vi "Construct_Remaining_Subtrack_101_More_2_Subtrks-1.vi"(0 "[IN] Still connected\ntracks in group":T2, 1 "[IN] Indexes for Jumps":i32[](array[numeric]), 5 "[IN] Clusters for Re\nconstructed Tracks":T1, 7 "[IN] Index of recon\nstructed tracks":i32, 11 "error IN":errorcluster, 12 "[IN] # column of re\nmaining elongation":i32, 13 "[IN] Indicies of Po\nints Inside Trks":i32[](array[numeric]), 14 "[IN] Indicies of all \nAffected Tracks \n(initial point = 0)":i32[](array[numeric])) -> (6 "[OUT] Clusters for Re\nconstructed Tracks":T1, 15 "error OUT":errorcluster)   [LabVIEW 2017]
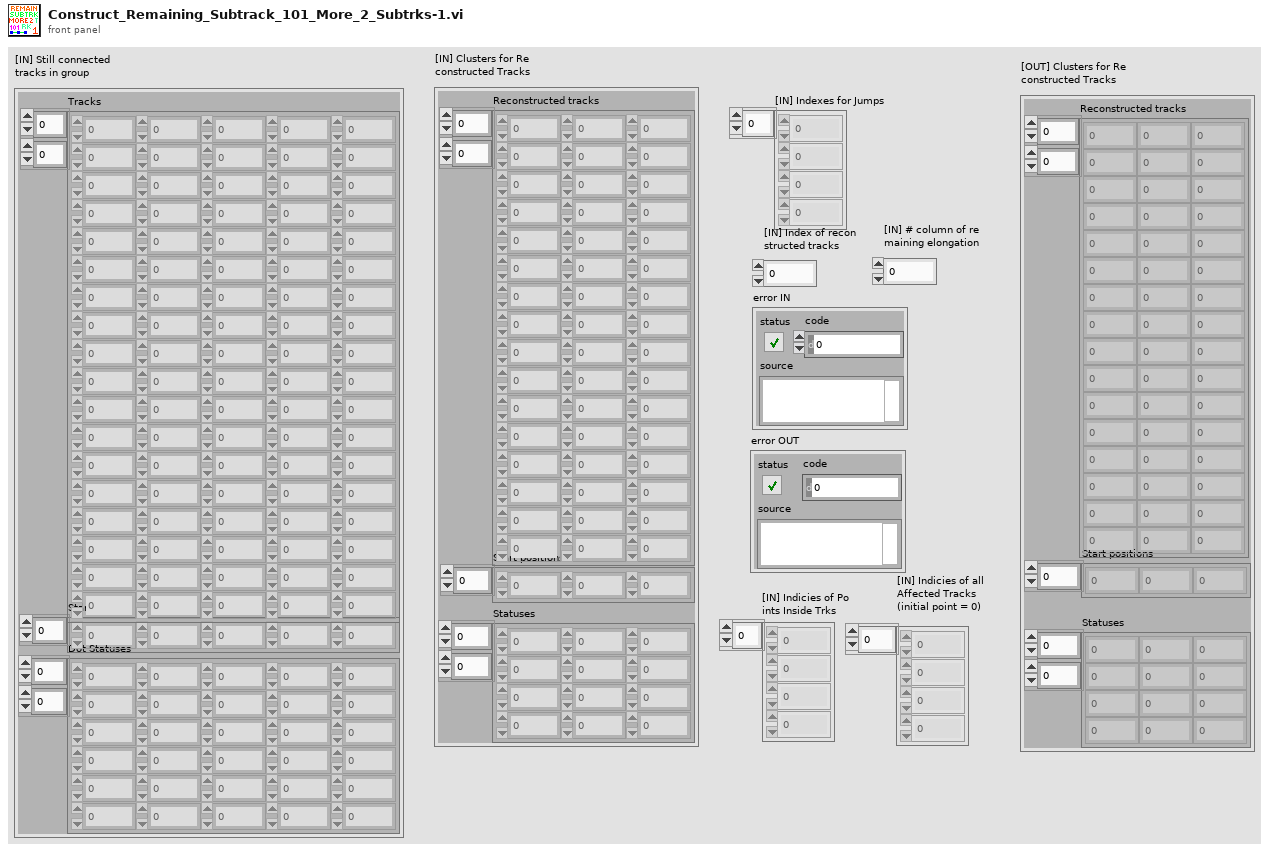
[diagram p1: front panel]
types:
  T1 = cluster{"Reconstructed tracks":dbl[][], "Start positions":i32[], "Statuses":i16[][]}
  T2 = cluster{"Tracks":dbl[][], "Start Pos":i32[], "Dot Statuses":i16[][]}
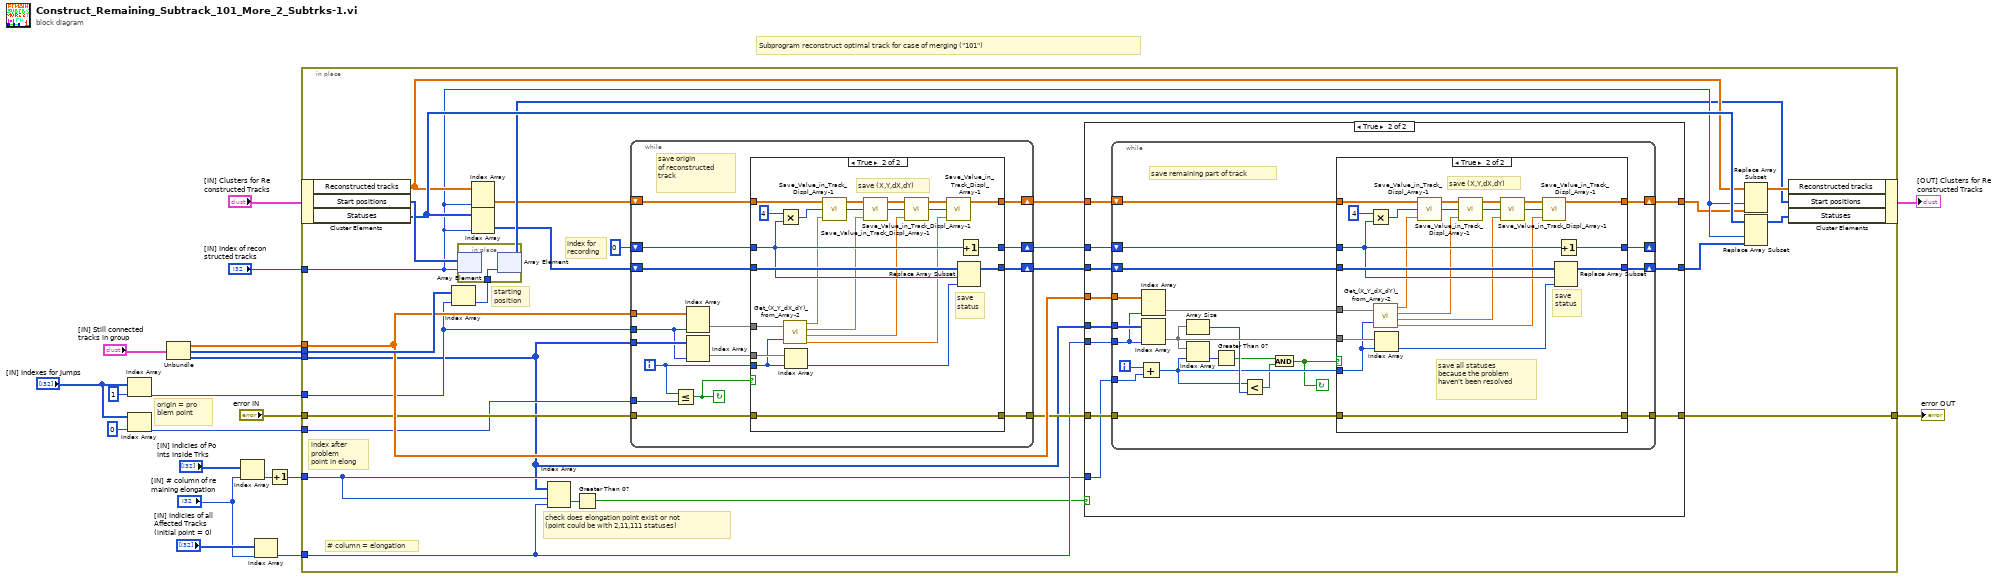
[diagram p0: block diagram]
diagram:
  # "origin = pro\nblem point"
  # "Subprogram reconstruct optimal track for case of merging (\"101\")"
  n1 = Index Array(array="[IN] Indexes for Jumps", index=1) -> (element=w14:i32)
  n2 = Index Array(array="[IN] Indexes for Jumps", index=0) -> (element=w10:i32)
  n3 = Unbundle("[IN] Still connected\ntracks in group") -> ("Tracks"=w11:dbl[][], "Start Pos"=w12:i32[], "Dot Statuses"=w13:i16[][])
  n4 = Index Array(array="[IN] Indicies of Po\nints Inside Trks", index="[IN] # column of re\nmaining elongation") -> (element=w3:i32)
  n5 = Index Array(array="[IN] Indicies of all \nAffected Tracks \n(initial point = 0)", index="[IN] # column of re\nmaining elongation") -> (element=w5:i32)
  n6 = Increment(x=w3) -> (x+1=w2:i32)
  n7 = in-place {
    in-place-border: "[IN] Index of recon\nstructed tracks" -> [w43]
    in-place-border: w14 -> [w25]
    in-place-border: w13 -> [w21]
    in-place-border: w12 -> [w48]
    in-place-border: w11 -> [w47]
    in-place-border: w10 -> [w24]
    in-place-border: "error IN" -> [w42]
    in-place-border: w5 -> [w27]
    in-place-border: [w38] -> w7
    in-place-border: w2 -> [w26]
    # "check does elongation point exist or not  \n(point could be with 2,11,111 statuses)"
    # "# column = elongation"
    # "index after\nproblem \npoint in elong"
    # "index for\nrecording"
    # "starting\nposition"
    n8 = in-place-cluster #1("[IN] Clusters for Re\nconstructed Tracks") -> ("Reconstructed tracks"=w44:dbl[][], "Start positions"=w46:i32[], "Statuses"=w45:i16[][])
    n9 = Index Array(array=w48, index=w25) -> (element=w37:i32)
    n10 = in-place {
      in-place-border: w37 -> [w154]
      n11 = in-place-array #2(w46, w43) -> ()  [unwired: 1 out]
      n12 = in-place-array #2(w154) -> (w40:i32[])  [unwired: 1 out]
    }
    n13 = Index Array(array=w44, index (col)=w43) -> (element=w35:dbl[])  [unwired: 1 in]
    n14 = Index Array(array=w45, index (col)=w43) -> (element=w34:i16[])  [unwired: 1 in]
    n15 = Index Array(array=w21, index (row)=w26, index (col)=w27) -> (element=w23:i16)
    n16 = Greater Than 0?(x=w23) -> (x > 0?=w22:bool)
    n17 = while {
      tunnel: w24 -> [w113]
      tunnel: w47 -> [w126]
      tunnel: w21 -> [w125]
      tunnel: w25 -> [w124]
      shift-right: [w118] -> w33
      shift-left: w35 -> [w123]
      shift-right: [w116] -> w31
      shift-left: w34 -> [w120]
      shift-right: [w117] -> w32
      shift-left: 0 -> [w119]
      tunnel: w42 -> [w111]
      tunnel: [w115] -> w30
      i -> [w114]
      stop <- w112 continue-if-true
      # "save origin \nof reconstructed \ntrack"
      n18 = Less Or Equal?(x=w114, y=w113) -> (x <= y?=w112:bool)
      n19 = Index Array(array=w126, index (col)=w124) -> (element=w122:dbl[])  [unwired: 1 in]
      n20 = Index Array(array=w125, index (col)=w124) -> (element=w121:i16[])  [unwired: 1 in]
      n21 = case shown="True" w112 {
        tunnel: w123 -> [w130 w143]
        tunnel: w122 -> [_ w153]
        tunnel: w121 -> [_ w152]
        tunnel: w114 -> [_ w148]
        tunnel: w120 -> [w128 w150]
        tunnel: [w128 w147] -> w116
        tunnel: [w130 w132] -> w118
        tunnel: w119 -> [w129 w146]
        tunnel: [w129 w145] -> w117
        tunnel: w111 -> [w127 w144]
        tunnel: [w127 w144] -> w115
        frame False {
        }
        frame True {
          # "save (X,Y,dX,dY)"
          # "save\nstatus"
          n22 = Multiply(x=4, y=w146) -> (x*y=w141:i32)
          n23 = call "Get_(X_Y_dX_dY)_from_Array-2.vi"("(X,Y,dX,dY)"=w153, "Index of Displacement"=w148) -> ("X"=w142:dbl, "Y"=w138:dbl, "dX"=w136:dbl, "dY"=w133:dbl)
          n24 = Index Array(array=w152, index=w148) -> (element=w149:i16)
          n25 = call "Save_Value_in_Track_Displ_Array-1.vi"("[IN] Value"=w142, "[IN] Index"=w141, "[IN] Empty tracks\nfor points saving"=w143) -> ("[OUT] Index ++"=w139:i32, "[OUT Track with saved value"=w140:dbl[])  [unwired: 1 in]
          n26 = call "Save_Value_in_Track_Displ_Array-1.vi"("[IN] Value"=w138, "[IN] Index"=w139, "[IN] Empty tracks\nfor points saving"=w140) -> ("[OUT] Index ++"=w135:i32, "[OUT Track with saved value"=w137:dbl[])  [unwired: 1 in]
          n27 = call "Save_Value_in_Track_Displ_Array-1.vi"("[IN] Value"=w136, "[IN] Index"=w135, "[IN] Empty tracks\nfor points saving"=w137) -> ("[OUT] Index ++"=w131:i32, "[OUT Track with saved value"=w134:dbl[])  [unwired: 1 in]
          n28 = call "Save_Value_in_Track_Displ_Array-1.vi"("[IN] Value"=w133, "[IN] Index"=w131, "[IN] Empty tracks\nfor points saving"=w134) -> ("[OUT Track with saved value"=w132:dbl[])  [unwired: 1 in, 1 out]
          n29 = Replace Array Subset(array=w150, new element=w149, index=w146) -> (w147:i16[])
          n30 = Increment(x=w146) -> (x+1=w145:i32)
        }
      }
    }
    n31 = case shown="True" w22 {
      tunnel: w47 -> [_ w62]
      tunnel: [w49 w61] -> w38
      tunnel: w33 -> [w51 w60]
      tunnel: w32 -> [_ w59]
      tunnel: w31 -> [w50 w58]
      tunnel: w30 -> [w49 w57]
      tunnel: [w51 w56] -> w29
      tunnel: [w50 w55] -> w28
      tunnel: w21 -> [_ w54]
      tunnel: w27 -> [_ w53]
      tunnel: w26 -> [_ w52]
      frame False {
      }
      frame True {
        n32 = while {
          tunnel: w62 -> [w83]
          tunnel: w54 -> [w82]
          tunnel: w53 -> [w81]
          shift-right: [w76] -> w56
          shift-left: w60 -> [w80]
          shift-right: [w74] -> w55
          shift-left: w58 -> [w78]
          shift-right: [w75] -> _
          shift-left: w59 -> [w77]
          tunnel: w52 -> [w72]
          tunnel: w57 -> [w64]
          tunnel: [w63] -> w61
          i -> [w73]
          stop <- w65 continue-if-true
          # "save remaining part of track"
          n33 = Add(x=w73, y=w72) -> (x+y=w68:i32)
          n34 = Index Array(array=w83, index (col)=w81) -> (element=w79:dbl[])  [unwired: 1 in]
          n35 = Index Array(array=w82, index (col)=w81) -> (element=w71:i16[])  [unwired: 1 in]
          n36 = Array Size(array=w71) -> (size(s)=w69:i32)
          n37 = Index Array(array=w71, index=w68) -> (element=w70:i16)
          n38 = Greater Than 0?(x=w70) -> (x > 0?=w67:bool)
          n39 = Less?(x=w68, y=w69) -> (x < y?=w66:bool)
          n40 = And(x=w67, y=w66) -> (x .and. y?=w65:bool)
          n41 = case shown="True" w65 {
            tunnel: w80 -> [w87 w101]
            tunnel: w79 -> [_ w110]
            tunnel: w71 -> [_ w109]
            tunnel: w68 -> [_ w102]
            tunnel: w78 -> [w85 w107]
            tunnel: [w85 w106] -> w74
            tunnel: [w87 w89] -> w76
            tunnel: w77 -> [w86 w105]
            tunnel: [w86 w104] -> w75
            tunnel: w64 -> [w84 w103]
            tunnel: [w84 w103] -> w63
            frame False {
            }
            frame True {
              # "save all statuses \nbecause the problem\nhaven't been resolved"
              # "save (X,Y,dX,dY)"
              # "save\nstatus"
              n42 = Multiply(x=4, y=w105) -> (x*y=w100:i32)
              n43 = call "Get_(X_Y_dX_dY)_from_Array-2.vi"("(X,Y,dX,dY)"=w110, "Index of Displacement"=w102) -> ("X"=w99:dbl, "Y"=w96:dbl, "dX"=w94:dbl, "dY"=w90:dbl)
              n44 = Index Array(array=w109, index=w102) -> (element=w88:i16)
              n45 = call "Save_Value_in_Track_Displ_Array-1.vi"("[IN] Value"=w99, "[IN] Index"=w100, "[IN] Empty tracks\nfor points saving"=w101) -> ("[OUT] Index ++"=w97:i32, "[OUT Track with saved value"=w98:dbl[])  [unwired: 1 in]
              n46 = call "Save_Value_in_Track_Displ_Array-1.vi"("[IN] Value"=w96, "[IN] Index"=w97, "[IN] Empty tracks\nfor points saving"=w98) -> ("[OUT] Index ++"=w93:i32, "[OUT Track with saved value"=w95:dbl[])  [unwired: 1 in]
              n47 = call "Save_Value_in_Track_Displ_Array-1.vi"("[IN] Value"=w94, "[IN] Index"=w93, "[IN] Empty tracks\nfor points saving"=w95) -> ("[OUT] Index ++"=w91:i32, "[OUT Track with saved value"=w92:dbl[])  [unwired: 1 in]
              n48 = call "Save_Value_in_Track_Displ_Array-1.vi"("[IN] Value"=w90, "[IN] Index"=w91, "[IN] Empty tracks\nfor points saving"=w92) -> ("[OUT Track with saved value"=w89:dbl[])  [unwired: 1 in, 1 out]
              n49 = Replace Array Subset(array=w107, new element=w88, index=w105) -> (w106:i16[])
              n50 = Increment(x=w105) -> (x+1=w104:i32)
            }
          }
        }
      }
    }
    n51 = Replace Array Subset(array=w44, new element=w29, index (col)=w43) -> (w41:dbl[][])  [unwired: 1 in]
    n52 = Replace Array Subset(array=w45, new element=w28, index (col)=w43) -> (w39:i16[][])  [unwired: 1 in]
    n53 = in-place-cluster #1("Reconstructed tracks"=w41, "Start positions"=w40, "Statuses"=w39) -> (→"[OUT] Clusters for Re\nconstructed Tracks":T1)
  }
  "error OUT" <- w7
